vi "Threshold Detector PtByPt.vi"(7 "initialize":bool, 9 "width":i32=1, 10 "threshold":dbl format="%0.2f", 11 "x":dbl format="%0.2f") -> (0 "error":i32, 2 "index":i32, 3 "detected":bool)   [LabVIEW 2020, in "NI_PtbyPt.lvlib"]
doc: "Analyzes the set of input data points specified by <B>width</B> for valid peaks and detects the set of points that exceed the <B>threshold</B> in a valid peak."
uses:
  <vilib>/ptbypt/NI_PtbyPt.lvlib
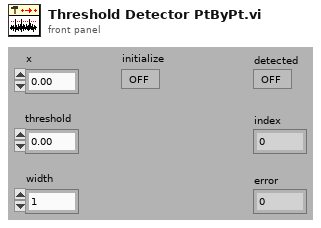
[diagram p1: front panel]
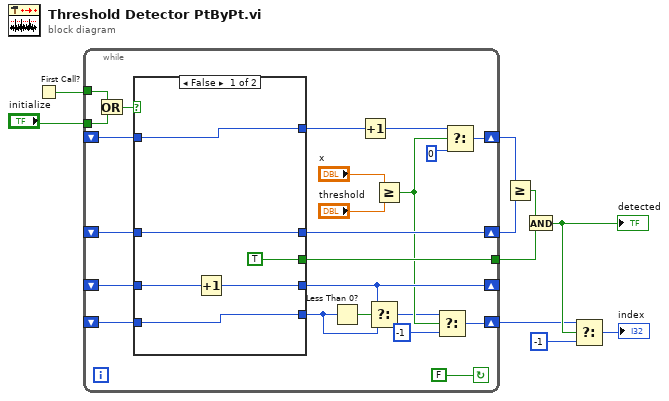
[diagram p0: block diagram]
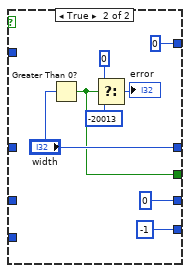
[diagram p2: hidden frame]
diagram:
  n1 = First Call?() -> (First Call?: T/F=w9:bool)
  n2 = while {
    tunnel: [w21] -> w6
    shift-left: _ -> [w28]
    shift-right: [w29] -> w8
    tunnel: w9 -> [w32]
    shift-left: _ -> [w30]
    shift-right: [w23] -> w10
    tunnel: "initialize" -> [w20]
    shift-right: [w15] -> _
    shift-left: _ -> [w19]
    shift-right: [w11] -> w3
    shift-left: _ -> [w18]
    stop <- FALSE continue-if-true
    n3 = Or(x=w32, y=w20) -> (x .or. y?=w31:bool)
    n4 = case shown="False" w31 {
      tunnel: [w35 0 ("f")] -> w24
      tunnel: w30 -> [w35 _]
      tunnel: [w39 "width"] -> w29
      tunnel: w28 -> [w39 _]
      tunnel: [TRUE w42] -> w21
      tunnel: [w36 0] -> w15
      tunnel: w19 -> [w37 _]
      tunnel: [w34 -1] -> w16
      tunnel: w18 -> [w34 _]
      frame False {
        n5 = Increment(x=w37) -> (x+1=w36:i32)
      }
      frame True {
        n6 = Greater Than 0?(x="width") -> (x > 0?=w42:bool)
        n7 = Select(t=0, s=w42, f=-20013) -> (s? t:f=→"error":i32)
      }
    }
    n8 = Less Than 0?(x=w16) -> (x < 0?=w17:bool)
    n9 = Increment(x=w24) -> (x+1=w22:i32)
    n10 = Select(t=w15, s=w17, f=w16) -> (s? t:f=w13:i32)
    n11 = Greater Or Equal?(x="x", y="threshold") -> (x >= y?=w14:bool)
    n12 = Select(t=w13, s=w14, f=-1) -> (s? t:f=w11:i32)
    n13 = Select(t=w22, s=w14, f=0) -> (s? t:f=w23:i32)
  }
  n14 = Greater Or Equal?(x=w10, y=w8) -> (x >= y?=w7:bool)
  n15 = And(x=w7, y=w6) -> (x .and. y?=w4:bool)
  "detected" <- w4
  n16 = Select(t=w3, s=w4, f=-1) -> (s? t:f=→"index":i32)
